vi "rsscope_core_global.vi"() -> ()   [LabVIEW 2014] (continued)
Name"="Protocol USB Trigger ET Check Max", "Data Type"=2, "Command"="TRIG{Trigger}:USB:TMAX", "Access"=2, "Range Table"="", "Read Callback"="", "Write Callback"="", "Supported Models"="", "Instrument Options"="K60", "Flags"=0, "Help"="Sets the end value of an endpoint type range if the corresponding condition is set to &apos;In range&apos; and &apos;Out of range&apos;.\n\nAvailable Repeated Capabilities:\nTrigger: TrigA, TrigB, TrigR\r\n\nRemote-control command(s):\nTRIGger<m>:USB:TMAX"}, {"Level"=2, "Class Only"=TRUE, "Identifier"="", "Descriptive Name"="USB 31 Generation 1", "Data Type"=0, "Command"="", "Access"=0, "Range Table"="", "Read Callback"="", "Write Callback"="", "Supported Models"="", "Instrument Options"="", "Flags"=0, "Help"="Configures USB 3.1 Generation 1 trigger."}, {"Level"=2, "Class Only"=TRUE, "Identifier"="", "Descriptive Name"="USB PD", "Data Type"=0, "Command"="", "Access"=0, "Range Table"="", "Read Callback"="", "Write Callback"="", "Supported Models"="", "Instrument Options"="", "Flags"=0, "Help"="Configures USB PD  trigger."}, {"Level"=3, "Class Only"=FALSE, "Identifier"="RSSCOPE_ATTR_USB_PD_TRIGGER_TYPE", "Descriptive Name"="USB PD Trigger Type", "Data Type"=0, "Command"="TRIG{Trigger}:USBP:TYPE", "Access"=2, "Range Table"="RsScope_rngUSBPDTriggerType", "Read Callback"="", "Write Callback"="", "Supported Models"="", "Instrument Options"="K63", "Flags"=0, "Help"="Selects the trigger type.\n\nAvailable Repeated Capabilities:\nTrigger: TrigA, TrigB, TrigR\r\n\nRemote-control command(s):\nTRIGger<m>:USBPd:TYPE"}, {"Level"=3, "Class Only"=FALSE, "Identifier"="RSSCOPE_ATTR_USB_PD_TRIGGER_PACKET_TYPE", "Descriptive Name"="USB PD Trigger Packet Type", "Data Type"=0, "Command"="TRIG{Trigger}:USBP:FRAM:SEL", "Access"=2, "Range Table"="RsScope_rngUSBPDPacketType", "Read Callback"="rsscope_empty_ReadCallback.vi", "Write Callback"="", "Supported Models"="", "Instrument Options"="K63", "Flags"=0, "Help"="Selects the frame to be triggered on, if the frame does not have any fields, e.g. a test frame.\n\nAvailable Repeated Capabilities:\nTrigger: TrigA, TrigB, TrigR\r\n\nRemote-control command(s):\nTRIGger<m>:USBPd:FRAMe:SELect"}, {"Level"=3, "Class Only"=TRUE, "Identifier"="", "Descriptive Name"="Data", "Data Type"=0, "Command"="", "Access"=0, "Range Table"="", "Read Callback"="", "Write Callback"="", "Supported Models"="", "Instrument Options"="", "Flags"=0, "Help"="Defines for the selected field, how a data check is executed."}, {"Level"=4, "Class Only"=FALSE, "Identifier"="RSSCOPE_ATTR_USB_PD_TRIGGER_DATA_CONDITION", "Descriptive Name"="USB PD Trigger Data Condition", "Data Type"=0, "Command"="TRIG{Trigger}:USBP:FRAM:FIEL{FieldNumber}:DOP", "Access"=2, "Range Table"="rsscope_rngProtocolTriggerCondition", "Read Callback"="rsscope_FormatUSBPDPacketTypeInt32_ReadCallback.vi", "Write Callback"="rsscope_FormatUSBPDPacketTypeInt32_WriteCallback.vi", "Supported Models"="", "Instrument Options"="K63", "Flags"=0, "Help"="Sets the condition for the data pattern. You can define no value, an exact value or a value range.\n\nAvailable Repeated Capabilities:\nTrigger: TrigA, TrigB, TrigR\r\nFieldNumber: Field1, Field2, Field3, Field4, Field5, Field6, Field7, Field8, Field9, Field10, Field11, Field12, Field13, Field14, Field15, Field16, Field17, Field18, Field19, Field20\r\n\nRemote-control command(s):\nTRIGger<m>:USBPd:FRAMe:FIELd<n>:DOPerator"}, {"Level"=4, "Class Only"=FALSE, "Identifier"="RSSCOPE_ATTR_USB_PD_TRIGGER_DATA_MIN", "Descriptive Name"="USB PD Trigger Data Min", "Data Type"=2, "Command"="TRIG{Trigger}:USBP:FRAM:FIEL{FieldNumber}:DMIN", "Access"=2, "Range Table"="", "Read Callback"="rsscope_FormatUSBPDPacketTypeString_ReadCallback.vi", "Write Callback"="rsscope_FormatUSBPDPacketTypeString_WriteCallback.vi", "Supported Models"="", "Instrument Options"="K63", "Flags"=0, "Help"="Specifies a data bit pattern, or sets the start value of a pattern range.\n\nValid Values:\nBinary pattern string consisting of 1; 0; or X (any bit).\n\nAvailable Repeated Capabilities:\nTrigger: TrigA, TrigB, TrigR\r\nFieldNumber: Field1, Field2, Field3, Field4, Field5, Field6, Field7, Field8, Field9, Field10, Field11, Field12, Field13, Field14, Field15, Field16, Field17, Field18, Field19, Field20\r\n\nRemote-control command(s):\nTRIGger<m>:USBPd:FRAMe:FIELd<n>:DMIN"}, {"Level"=4, "Class Only"=FALSE, "Identifier"="RSSCOPE_ATTR_USB_PD_TRIGGER_DATA_MAX", "Descriptive Name"="USB PD Trigger Data Max", "Data Type"=2, "Command"="TRIG{Trigger}:USBP:FRAM:FIEL{FieldNumber}:DMAX", "Access"=2, "Range Table"="", "Read Callback"="rsscope_FormatUSBPDPacketTypeString_ReadCallback.vi", "Write Callback"="rsscope_FormatUSBPDPacketTypeString_WriteCallback.vi", "Supported Models"="", "Instrument Options"="K63", "Flags"=0, "Help"="Sets the end value of a data type range for condition In Range or Out of Range. \n\nValid Values:\nBinary pattern string consisting of 1; 0; or X (any bit).\n\nAvailable Repeated Capabilities:\nTrigger: TrigA, TrigB, TrigR\r\nFieldNumber: Field1, Field2, Field3, Field4, Field5, Field6, Field7, Field8, Field9, Field10, Field11, Field12, Field13, Field14, Field15, Field16, Field17, Field18, Field19, Field20\r\n\nRemote-control command(s):\nTRIGger<m>:USBPd:FRAMe:FIELd<n>:DMAX"}, {"Level"=3, "Class Only"=TRUE, "Identifier"="", "Descriptive Name"="Index", "Data Type"=0, "Command"="", "Access"=0, "Range Table"="", "Read Callback"="", "Write Callback"="", "Supported Models"="", "Instrument Options"="", "Flags"=0, "Help"="Defines for the selected field, how an index check is executed."}, {"Level"=4, "Class Only"=FALSE, "Identifier"="RSSCOPE_ATTR_USB_PD_TRIGGER_INDEX_CONDITION", "Descriptive Name"="USB PD Trigger Index Condition", "Data Type"=0, "Command"="TRIG{Trigger}:USBP:FRAM:FIEL{FieldNumber}:IOP", "Access"=2, "Range Table"="rsscope_rngUSB31Gen1IndexCondition", "Read Callback"="rsscope_FormatUSBPDPacketTypeInt32_ReadCallback.vi", "Write Callback"="rsscope_FormatUSBPDPacketTypeInt32_WriteCallback.vi", "Supported Models"="", "Instrument Options"="K63", "Flags"=0, "Help"="Sets the operator for the index in the selected field of the selected frame.\n\nAvailable Repeated Capabilities:\nTrigger: TrigA, TrigB, TrigR\r\nFieldNumber: Field1, Field2, Field3, Field4, Field5, Field6, Field7, Field8, Field9, Field10, Field11, Field12, Field13, Field14, Field15, Field16, Field17, Field18, Field19, Field20\r\n\nRemote-control command(s):\nTRIGger<m>:USBPd:FRAMe:FIELd<n>:IOPerator"}, {"Level"=4, "Class Only"=FALSE, "Identifier"="RSSCOPE_ATTR_USB_PD_TRIGGER_INDEX_MIN", "Descriptive Name"="USB PD Trigger Index Min", "Data Type"=0, "Command"="TRIG{Trigger}:USBP:FRAM:FIEL{FieldNumber}:IMIN", "Access"=2, "Range Table"="", "Read Callback"="rsscope_FormatUSBPDPacketTypeInt32_ReadCallback.vi", "Write Callback"="rsscope_FormatUSBPDPacketTypeInt32_WriteCallback.vi", "Supported Models"="", "Instrument Options"="K63", "Flags"=0, "Help"="Specifies a data bit pattern, or sets the start value of a pattern range.\n\nValid Values:\nBinary pattern string consisting of 1; 0; or X (any bit).\n\nAvailable Repeated Capabilities:\nTrigger: TrigA, TrigB, TrigR\r\nFieldNumber: Field1, Field2, Field3, Field4, Field5, Field6, Field7, Field8, Field9, Field10, Field11, Field12, Field13, Field14, Field15, Field16, Field17, Field18, Field19, Field20\r\n\nRemote-control command(s):\nTRIGger<m>:USBPd:FRAMe:FIELd<n>:IMIN"}, {"Level"=4, "Class Only"=FALSE, "Identifier"="RSSCOPE_ATTR_USB_PD_TRIGGER_INDEX_MAX", "Descriptive Name"="USB PD Trigger Index Max", "Data Type"=0, "Command"="TRIG{Trigger}:USBP:FRAM:FIEL{FieldNumber}:IMAX", "Access"=2, "Range Table"="", "Read Callback"="rsscope_FormatUSBPDPacketTypeInt32_ReadCallback.vi", "Write Callback"="rsscope_FormatUSBPDPacketTypeInt32_WriteCallback.vi", "Supported Models"="", "Instrument Options"="K63", "Flags"=0, "Help"="Sets the end value of a data type range for condition In Range or Out of Range. \n\nValid Values:\nBinary pattern string consisting of 1; 0; or X (any bit).\n\nAvailable Repeated Capabilities:\nTrigger: TrigA, TrigB, TrigR\r\nFieldNumber: Field1, Field2, Field3, Field4, Field5, Field6, Field7, Field8, Field9, Field10, Field11, Field12, Field13, Field14, Field15, Field16, Field17, Field18, Field19, Field20\r\n\nRemote-control command(s):\nTRIGger<m>:USBPd:FRAMe:FIELd<n>:IMAX"}, {"Level"=3, "Class Only"=TRUE, "Identifier"="", "Descriptive Name"="Bit State", "Data Type"=0, "Command"="", "Access"=0, "Range Table"="", "Read Callback"="", "Write Callback"="", "Supported Models"="", "Instrument Options"="", "Flags"=0, "Help"="Defines the bit state to be checked for the selected field. Permitted bit states are 1, 0 or X (don&apos;t care)."}, {"Level"=4, "Class Only"=FALSE, "Identifier"="RSSCOPE_ATTR_USB_PD_TRIGGER_BIT_STATE", "Descriptive Name"="USB PD Trigger Bit State", "Data Type"=0, "Command"="TRIG{Trigger}:USBP:FRAM:FIEL{FieldNumber}:BIT", "Access"=2, "Range Table"="RsScope_rngBitState", "Read Callback"="rsscope_FormatUSBPDPacketTypeInt32_ReadCallback.vi", "Write Callback"="rsscope_FormatUSBPDPacketTypeInt32_WriteCallback.vi", "Supported Models"="", "Instrument Options"="K63", "Flags"=0, "Help"="Sets the bit state of a field that only consists of one bit.\n\nAvailable Repeated Capabilities:\nTrigger: TrigA, TrigB, TrigR\r\nFieldNumber: Field1, Field2, Field3, Field4, Field5, Field6, Field7, Field8, Field9, Field10, Field11, Field12, Field13, Field14, Field15, Field16, Field17, Field18, Field19, Field20\r\n\nRemote-control command(s):\nTRIGger<m>:USBPd:FRAMe:FIELd<n>:BIT"}, {"Level"=2, "Class Only"=TRUE, "Identifier"="", "Descriptive Name"="Custom Manchester NRZ", "Data Type"=0, "Command"="", "Access"=0, "Range Table"="", "Read Callback"="", "Write Callback"="", "Supported Models"="", "Instrument Options"="", "Flags"=0, "Help"="R&S RTO-K50 is a firmware option that enables the R&S RTO to analyze customizable serial bus signals encoded by the following coding standards: Manchester, Manchester II, NRZ Clocked, NRZ Unclocked."}, {"Level"=3, "Class Only"=FALSE, "Identifier"="RSSCOPE_ATTR_MANCHESTER_NRZ_TRIGGER_TYPE", "Descriptive Name"="Manchester NRZ Trigger Type", "Data Type"=0, "Command"="TRIG{Trigger}:CMSB:TYPE", "Access"=2, "Range Table"="RsScope_rngTriggerManchesterNRZType", "Read Callback"="", "Write Callback"="", "Supported Models"="", "Instrument Options"="K50", "Flags"=0, "Help"="Selects the trigger type for custom serial bus analysis.\n\nAvailable Repeated Capabilities:\nTrigger: TrigA, TrigB, TrigR\r\n\nRemote-control command(s):\nTRIGger<m>:CMSB:TYPE"}, {"Level"=3, "Class Only"=FALSE, "Identifier"="RSSCOPE_ATTR_MANCHESTER_NRZ_TRIGGER_DATA_PATTERN", "Descriptive Name"="Manchester NRZ Trigger Data Pattern", "Data Type"=2, "Command"="TRIG{Trigger}:CMSB:PATT", "Access"=2, "Range Table"="", "Read Callback"="", "Write Callback"="", "Supported Models"="", "Instrument Options"="K50", "Flags"=0, "Help"="Sets the pattern match conditions for a payload data check. The trigger is set to the first occurrence of a matching data bit pattern (which can be freely specified), starting after the minimum gap time and after the detected start of the data frame.\n\nAvailable Repeated Capabilities:\nTrigger: TrigA, TrigB, TrigR\r\n\nRemote-control command(s):\nTRIGger<m>:CMSB:PATTern"}, {"Level"=3, "Class Only"=FALSE, "Identifier"="RSSCOPE_ATTR_MANCHESTER_NRZ_TRIGGER_INDEX_CONDITION", "Descriptive Name"="Manchester NRZ Trigger Index Condition", "Data Type"=0, "Command"="TRIG{Trigger}:CMSB:ICON", "Access"=2, "Range Table"="rsscope_rngProtocolDataIndexOperator", "Read Callback"="", "Write Callback"="", "Supported Models"="", "Instrument Options"="K50", "Flags"=0, "Help"="Sets the operator to set a specific bit index (data position).\n\nAvailable Repeated Capabilities:\nTrigger: TrigA, TrigB, TrigR\r\n\nRemote-control command(s):\nTRIGger<m>:CMSB:ICONdition"}, {"Level"=3, "Class Only"=FALSE, "Identifier"="RSSCOPE_ATTR_MANCHESTER_NRZ_TRIGGER_INDEX_MIN", "Descriptive Name"="Manchester NRZ Trigger Index Min", "Data Type"=0, "Command"="TRIG{Trigger}:CMSB:IMIN", "Access"=2, "Range Table"="RsScope_rngManchesterNRZTriggerIndex", "Read Callback"="", "Write Callback"="", "Supported Models"="", "Instrument Options"="K50", "Flags"=0, "Help"="Sets the bit index (data position). If Index Condition is set to IN Range, IndexMin sets the start value of the bit index range.\n\nAvailable Repeated Capabilities:\nTrigger: TrigA, TrigB, TrigR\r\n\nRemote-control command(s):\nTRIGger<m>:CMSB:IMIN"}, {"Level"=3, "Class Only"=FALSE, "Identifier"="RSSCOPE_ATTR_MANCHESTER_NRZ_TRIGGER_INDEX_MAX", "Descriptive Name"="Manchester NRZ Trigger Index Max", "Data Type"=0, "Command"="TRIG{Trigger}:CMSB:IMAX", "Access"=2, "Range Table"="RsScope_rngManchesterNRZTriggerIndex", "Read Callback"="", "Write Callback"="", "Supported Models"="", "Instrument Options"="", "Flags"=0, "Help"="Sets the end value of the bit index range (data position range), if condition is set to In Range.\n\nAvailable Repeated Capabilities:\nTrigger: TrigA, TrigB, TrigR\r\n\nRemote-control command(s):\nTRIGger<m>:CMSB:IMAX"}, {"Level"=3, "Class Only"=FALSE, "Identifier"="RSSCOPE_ATTR_NRZ_TRIGGER_WORD_LENGTH", "Descriptive Name"="NRZ Trigger Word Length", "Data Type"=0, "Command"="TRIG{Trigger}:CMSB:NRZ:WRDL", "Access"=2, "Range Table"="RsScope_rngNRZTriggerWordLength", "Read Callback"="", "Write Callback"="", "Supported Models"="", "Instrument Options"="K50", "Flags"=0, "Help"="Sets the number of bits in an NRZ unclocked word.\n\nAvailable Repeated Capabilities:\nTrigger: TrigA, TrigB, TrigR\r\n\nRemote-control command(s):\nTRIGger<m>:CMSB:NRZ:WRDLength"}, {"Level"=2, "Class Only"=TRUE, "Identifier"="", "Descriptive Name"="SENT", "Data Type"=0, "Command"="", "Access"=0, "Range Table"="", "Read Callback"="", "Write Callback"="", "Supported Models"="", "Instrument Options"="", "Flags"=0, "Help"="SENT (Single Ended Nibble Transmission, R&S RTO-K10 option) is a serial transmission interface protocol originally specified for the communication of sensors and control units in automotive electronics."}, {"Level"=3, "Class Only"=FALSE, "Identifier"="RSSCOPE_ATTR_SENT_TRIGGER_TYPE", "Descriptive Name"="SENT Trigger Type", "Data Type"=0, "Command"="TRIG{Trigger}:SENT:TYPE", "Access"=2, "Range Table"="RsScope_rngSENTTriggerType", "Read Callback"="", "Write Callback"="", "Supported Models"="", "Instrument Options"="K10", "Flags"=0, "Help"="Selects the trigger event for the SENT transmission type.\n\nAvailable Repeated Capabilities:\nTrigger: TrigA, TrigB, TrigR\r\n\nRemote-control command(s):\nTRIGger<m>:SENT:TYPE"}, {"Level"=3, "Class Only"=TRUE, "Identifier"="", "Descriptive Name"="Transmission Sequence", "Data Type"=0, "Command"="", "Access"=0, "Range Table"="", "Read Callback"="", "Write Callback"="", "Supported Models"="", "Instrument Options"="", "Flags"=0, "Help"="Configures the trigger conditions for trigger type transmission sequence."}, {"Level"=4, "Class Only"=FALSE, "Identifier"="RSSCOPE_ATTR_SENT_TRIGGER_TRANSMISSION_SEQUENCE_TYPE", "Descriptive Name"="SENT Trigger Transmission Sequence Type", "Data Type"=0, "Command"="TRIG{Trigger}:SENT:TTYP", "Access"=2, "Range Table"="RsScope_rngSENTTriggerTSType", "Read Callback"="", "Write Callback"="", "Supported Models"="", "Instrument Options"="K10", "Flags"=0, "Help"="Selects the trigger event for the SENT transmission type.\n\nAvailable Repeated Capabilities:\nTrigger: TrigA, TrigB, TrigR\r\n\nRemote-control command(s):\nTRIGger<m>:SENT:TTYPe"}, {"Level"=4, "Class Only"=FALSE, "Identifier"="RSSCOPE_ATTR_SENT_TRIGGER_TRANSMISSION_SEQUENCE_STATUS", "Descriptive Name"="SENT Trigger Transmission Sequence Status", "Data Type"=2, "Command"="TRIG{Trigger}:SENT:STAT", "Access"=2, "Range Table"="", "Read Callback"="", "Write Callback"="", "Supported Models"="", "Instrument Options"="K10", "Flags"=0, "Help"="Sets the status nibble data, numeric or string pattern. The string parameter accepts the bit value X (don&apos;t care).\n\nAvailable Repeated Capabilities:\nTrigger: TrigA, TrigB, TrigR\r\n\nRemote-control command(s):\nTRIGger<m>:SENT:STATus"}, {"Level"=4, "Class Only"=FALSE, "Identifier"="RSSCOPE_ATTR_SENT_TRIGGER_TRANSMISSION_SEQUENCE_CONDITION", "Descriptive Name"="SENT Trigger Transmission Sequence Condition", "Data Type"=0, "Command"="TRIG{Trigger}:SENT:TDCN", "Access"=2, "Range Table"="rsscope_rngProtocolTriggerCondition", "Read Callback"="", "Write Callback"="", "Supported Models"="", "Instrument Options"="K10", "Flags"=0, "Help"="Sets the operator to set a specific data pattern or a data pattern range.\n\nAvailable Repeated Capabilities:\nTrigger: TrigA, TrigB, TrigR\r\n\nRemote-control command(s):\nTRIGger<m>:SENT:TDCN"}, {"Level"=4, "Class Only"=FALSE, "Identifier"="RSSCOPE_ATTR_SENT_TRIGGER_TRANSMISSION_SEQUENCE_DATA_MIN", "Descriptive Name"="SENT Trigger Transmission Sequence Data Min", "Data Type"=2, "Command"="TRIG{Trigger}:SENT:TDMN", "Access"=2, "Range Table"="", "Read Callback"="", "Write Callback"="", "Supported Models"="", "Instrument Options"="K10", "Flags"=0, "Help"="Specifies a data pattern, or sets the start value of a data pattern range. \n\nValid Values:\nBinary pattern string consisting of 1; 0; or X (any bit).\n\nAvailable Repeated Capabilities:\nTrigger: TrigA, TrigB, TrigR\r\n\nRemote-control command(s):\nTRIGger<m>:SENT:TDMN"}, {"Level"=4, "Class Only"=FALSE, "Identifier"="RSSCOPE_ATTR_SENT_TRIGGER_TRANSMISSION_SEQUENCE_DATA_MAX", "Descriptive Name"="SENT Trigger Transmission Sequence Data Max", "Data Type"=2, "Command"="TRIG{Trigger}:SENT:TDMX", "Access"=2, "Range Table"="", "Read Callback"="", "Write Callback"="", "Supported Models"="", "Instrument Options"="K10", "Flags"=0, "Help"="Sets the end value of an identifier range for condition In Range or Out of Range. \n\nValid Values:\nBinary pattern string consisting of 1; 0; or X (any bit).\n\nAvailable Repeated Capabilities:\nTrigger: TrigA, TrigB, TrigR\r\n\nRemote-control command(s):\nTRIGger<m>:SENT:TDMX"}, {"Level"=3, "Class Only"=TRUE, "Identifier"="", "Descriptive Name"="Serial Message", "Data Type"=0, "Command"="", "Access"=0, "Range Table"="", "Read Callback"="", "Write Callback"="", "Supported Models"="", "Instrument Options"="", "Flags"=0, "Help"="Configures the trigger conditions for a serial message."}, {"Level"=4, "Class Only"=FALSE, "Identifier"="RSSCOPE_ATTR_SENT_TRIGGER_SERIAL_MESSAGE_TYPE", "Descriptive Name"="SENT Trigger Serial Message Type", "Data Type"=0, "Command"="TRIG{Trigger}:SENT:STYP", "Access"=2, "Range Table"="RsScope_rngSENTTriggerSMType", "Read Callback"="", "Write Callback"="", "Supported Models"="", "Instrument Options"="K10", "Flags"=0, "Help"="Selects the trigger event for the serial message.\n\nAvailable Repeated Capabilities:\nTrigger: TrigA, TrigB, TrigR\r\n\nRemote-control command(s):\nTRIGger<m>:SENT:STYPe"}, {"Level"=4, "Class Only"=FALSE, "Identifier"="RSSCOPE_ATTR_SENT_TRIGGER_SERIAL_MESSAGE_ID_TYPE", "Descriptive Name"="SENT Trigger Serial Message ID Type", "Data Type"=0, "Command"="TRIG{Trigger}:SENT:SIDT", "Access"=2, "Range Table"="RsScope_rngSENTIDType", "Read Callback"="", "Write Callback"="", "Supported Models"="", "Instrument Options"="K10", "Flags"=0, "Help"="Sets the message ID format (4 bit or 8 bit) of the enhanced serial message.\n\nAvailable Repeated Capabilities:\nTrigger: TrigA, TrigB, TrigR\r\n\nRemote-control command(s):\nTRIGger<m>:SENT:SIDType"}, {"Level"=4, "Class Only"=FALSE, "Identifier"="RSSCOPE_ATTR_SENT_TRIGGER_SERIAL_MESSAGE_ID_CONDITION", "Descriptive Name"="SENT Trigger Serial Message ID Condition", "Data Type"=0, "Command"="TRIG{Trigger}:SENT:SICN", "Access"=2, "Range Table"="rsscope_rngProtocolTriggerCondition", "Read Callback"="", "Write Callback"="", "Supported Models"="", "Instrument Options"="K10", "Flags"=0, "Help"="Sets the operator to set a specific data pattern or a data pattern range.\n\nAvailable Repeated Capabilities:\nTrigger: TrigA, TrigB, TrigR\r\n\nRemote-control command(s):\nTRIGger<m>:SENT:SICN"}, {"Level"=4, "Class Only"=FALSE, "Identifier"="RSSCOPE_ATTR_SENT_TRIGGER_SERIAL_MESSAGE_ID_MIN", "Descriptive Name"="SENT Trigger Serial Message ID Min", "Data Type"=2, "Command"="TRIG{Trigger}:SENT:SIMN", "Access"=2, "Range Table"="", "Read Callback"="", "Write Callback"="", "Supported Models"="", "Instrument Options"="K10", "Flags"=0, "Help"="Specifies a message identifier pattern, or sets the start value of an identifier range. \n\nValid Values:\nBinary pattern string consisting of 1; 0; or X (any bit).\n\nAvailable Repeated Capabilities:\nTrigger: TrigA, TrigB, TrigR\r\n\nRemote-control command(s):\nTRIGger<m>:SENT:SIMN"}, {"Level"=4, "Class Only"=FALSE, "Identifier"="RSSCOPE_ATTR_SENT_TRIGGER_SERIAL_MESSAGE_ID_MAX", "Descriptive Name"="SENT Trigger Serial Message ID Max", "Data Type"=2, "Command"="TRIG{Trigger}:SENT:SIMX", "Access"=2, "Range Table"="", "Read Callback"="", "Write Callback"="", "Supported Models"="", "Instrument Options"="K10", "Flags"=0, "Help"="Sets the end value of an identifier range for condition In Range or Out of Range.\n\nValid Values:\nBinary pattern string consisting of 1; 0; or X (any bit).\n\nAvailable Repeated Capabilities:\nTrigger: TrigA, TrigB, TrigR\r\n\nRemote-control command(s):\nTRIGger<m>:SENT:SIMX"}, {"Level"=4, "Class Only"=FALSE, "Identifier"="RSSCOPE_ATTR_SENT_TRIGGER_SERIAL_MESSAGE_DATA_CONDITION", "Descriptive Name"="SENT Trigger Serial Message Data Condition", "Data Type"=0, "Command"="TRIG{Trigger}:SENT:SDCN", "Access"=2, "Range Table"="rsscope_rngProtocolTriggerCondition", "Read Callback"="", "Write Callback"="", "Supported Models"="", "Instrument Options"="K10", "Flags"=0, "Help"="Sets the operator to define a specific data pattern or a data pattern range.\n\nAvailable Repeated Capabilities:\nTrigger: TrigA, TrigB, TrigR\r\n\nRemote-control command(s):\nTRIGger<m>:SENT:SDCN"}, {"Level"=4, "Class Only"=FALSE, "Identifier"="RSSCOPE_ATTR_SENT_TRIGGER_SERIAL_MESSAGE_DATA_MIN", "Descriptive Name"="SENT Trigger Serial Message Data Min", "Data Type"=2, "Command"="TRIG{Trigger}:SENT:SDMN", "Access"=2, "Range Table"="", "Read Callback"="", "Write Callback"="", "Supported Models"="", "Instrument Options"="K10", "Flags"=0, "Help"="Specifies a data pattern, or sets the start value of a data pattern range.\n\nValid Values:\nBinary pattern string consisting of 1; 0; or X (any bit).\n\nAvailable Repeated Capabilities:\nTrigger: TrigA, TrigB, TrigR\r\n\nRemote-control command(s):\nTRIGger<m>:SENT:SDMN"}, {"Level"=4, "Class Only"=FALSE, "Identifier"="RSSCOPE_ATTR_SENT_TRIGGER_SERIAL_MESSAGE_DATA_MAX", "Descriptive Name"="SENT Trigger Serial Message Data Max", "Data Type"=2, "Command"="TRIG{Trigger}:SENT:SDMX", "Access"=2, "Range Table"="", "Read Callback"="", "Write Callback"="", "Supported Models"="", "Instrument Options"="K10", "Flags"=0, "Help"="Sets the end value of an identifier range for condition In Range or Out of Range.\n\nValid Values:\nBinary pattern string consisting of 1; 0; or X (any bit).\n\nAvailable Repeated Capabilities:\nTrigger: TrigA, TrigB, TrigR\r\n\nRemote-control command(s):\nTRIGger<m>:SENT:SDMX"}, {"Level"=3, "Class Only"=TRUE, "Identifier"="", "Descriptive Name"="Error Conditions", "Data Type"=0, "Command"="", "Access"=0, "Range Table"="", "Read Callback"="", "Write Callback"="", "Supported Models"="", "Instrument Options"="", "Flags"=0, "Help"="This class configures conditions for Error trigger."}, {"Level"=4, "Class Only"=FALSE, "Identifier"="RSSCOPE_ATTR_PROTOCOL_SENT_TRIGGER_FORM_ERROR", "Descriptive Name"="Protocol SENT Trigger Form Error", "Data Type"=3, "Command"="TRIG{Trigger}:SENT:FORM", "Access"=2, "Range Table"="", "Read Callback"="", "Write Callback"="", "Supported Models"="", "Instrument Options"="K10", "Flags"=0, "Help"="Triggers on format errors in serial messages.\n\nAvailable Repeated Capabilities:\nTrigger: TrigA, TrigB, TrigR\r\n\nRemote-control command(s):\nTRIGger<m>:SENT:FORMerror"}, {"Level"=4, "Class Only"=FALSE, "Identifier"="RSSCOPE_ATTR_PROTOCOL_SENT_TRIGGER_CALIBRATION_PULSE_ERROR", "Descriptive Name"="Protocol SENT Trigger Calibration Pulse Error", "Data Type"=3, "Command"="TRIG{Trigger}:SENT:PULS", "Access"=2, "Range Table"="", "Read Callback"="", "Write Callback"="", "Supported Models"="", "Instrument Options"="K10", "Flags"=0, "Help"="Triggers on calibration pulse erors in transmission sequences.\n\nAvailable Repeated Capabilities:\nTrigger: TrigA, TrigB, TrigR\r\n\nRemote-control command(s):\nTRIGger<m>:SENT:PULSeerror"}, {"Level"=4, "Class Only"=FALSE, "Identifier"="RSSCOPE_ATTR_PROTOCOL_SENT_TRIGGER_PULSE_PERIOD_ERROR", "Descriptive Name"="Protocol SENT Trigger Pulse Period Error", "Data Type"=3, "Command"="TRIG{Trigger}:SENT:PPER", "Access"=2, "Range Table"="", "Read Callback"="", "Write Callback"="", "Supported Models"="", "Instrument Options"="K10", "Flags"=0, "Help"="Triggers on pulse period errors.\n\nAvailable Repeated Capabilities:\nTrigger: TrigA, TrigB, TrigR\r\n\nRemote-control command(s):\nTRIGger<m>:SENT:PPERioderror"}, {"Level"=4, "Class Only"=FALSE, "Identifier"="RSSCOPE_ATTR_PROTOCOL_SENT_TRIGGER_CRC_ERROR", "Descriptive Name"="Protocol SENT Trigger CRC Error", "Data Type"=3, "Command"="TRIG{Trigger}:SENT:CRC", "Access"=2, "Range Table"="", "Read Callback"="", "Write Callback"="", "Supported Models"="", "Instrument Options"="K10", "Flags"=0, "Help"="Triggers on CRC errors in both, the transmission sequences and serial messages.\n\nAvailable Repeated Capabilities:\nTrigger: TrigA, TrigB, TrigR\r\n\nRemote-control command(s):\nTRIGger<m>:SENT:CRCerror"}, {"Level"=4, "Class Only"=FALSE, "Identifier"="RSSCOPE_ATTR_PROTOCOL_SENT_TRIGGER_IRREGULAR_FRAME_LENGTH_ERROR", "Descriptive Name"="Protocol SENT Trigger Irregular Frame Length Error", "Data Type"=3, "Command"="TRIG{Trigger}:SENT:IRFL", "Access"=2, "Range Table"="", "Read Callback"="", "Write Callback"="", "Supported Models"="", "Instrument Options"="K10", "Flags"=0, "Help"="Triggers on frame length errors in transmission sequences when pause pulse for constant frame length is set.\n\nAvailable Repeated Capabilities:\nTrigger: TrigA, TrigB, TrigR\r\n\nRemote-control command(s):\nTRIGger<m>:SENT:IRFLength"}, {"Level"=2, "Class Only"=TRUE, "Identifier"="", "Descriptive Name"="D-PHY", "Data Type"=0, "Command"="", "Access"=0, "Range Table"="", "Read Callback"="", "Write Callback"="", "Supported Models"="", "Instrument Options"="", "Flags"=0, "Help"="In this class all trigger settings can be configured."}, {"Level"=3, "Class Only"=FALSE, "Identifier"="RSSCOPE_ATTR_DPHY_TRIGGER_TYPE", "Descriptive Name"="DPHY Trigger Type", "Data Type"=0, "Command"="TRIG{Trigger}:DPHY:TYPE", "Access"=2, "Range Table"="RsScope_rngDPHYTriggerType", "Read Callback"="", "Write Callback"="", "Supported Models"="", "Instrument Options"="K42", "Flags"=0, "Help"="Sets the type of frame to be triggered on.\n\nAvailable Repeated Capabilities:\nTrigger: TrigA, TrigB, TrigR\r\n\nRemote-control command(s):\nTRIGger<m>:DPHY:TYPE"}, {"Level"=3, "Class Only"=FALSE, "Identifier"="RSSCOPE_ATTR_DPHY_TRIGGER_VIRTUAL_CHANNEL", "Descriptive Name"="DPHY Trigger Virtual Channel", "Data Type"=2, "Command"="TRIG{Trigger}:DPHY:HSVC", "Access"=2, "Range Table"="", "Read Callback"="", "Write Callback"="", "Supported Models"="", "Instrument Options"="K42", "Flags"=0, "Help"="Sets the virtual channel to be triggered on.\n\nAvailable Repeated Capabilities:\nTrigger: TrigA, TrigB, TrigR\r\n\nRemote-control command(s):\nTRIGger<m>:DPHY:HSVC"}, {"Level"=3, "Class Only"=TRUE, "Identifier"="", "Descriptive Name"="Data Type", "Data Type"=0, "Command"="", "Access"=0, "Range Table"="", "Read Callback"="", "Write Callback"="", "Supported Models"="", "Instrument Options"="", "Flags"=0, "Help"="Sets the specified data type to be triggered on. The data type setup consists of the condition and one or two data patterns."}, {"Level"=4, "Class Only"=FALSE, "Identifier"="RSSCOPE_ATTR_DPHY_TRIGGER_DATA_TYPE_CONDITION", "Descriptive Name"="DPHY Trigger Data Type Condition", "Data Type"=0, "Command"="TRIG{Trigger}:DPHY:DTYP:COND", "Access"=2, "Range Table"="rsscope_rngProtocolTriggerCondition", "Read Callback"="", "Write Callback"="", "Supported Models"="", "Instrument Options"="K42", "Flags"=0, "Help"="Set the condition for the data type. You can define an exact value or a value range.\n\nAvailable Repeated Capabilities:\nTrigger: TrigA, TrigB, TrigR\r\n\nRemote-control command(s):\nTRIGger<m>:DPHY:DTYPe:CONDition"}, {"Level"=4, "Class Only"=FALSE, "Identifier"="RSSCOPE_ATTR_DPHY_TRIGGER_DATA_TYPE_MIN", "Descriptive Name"="DPHY Trigger Data Type Min", "Data Type"=2, "Command"="TRIG{Trigger}:DPHY:DTYP:MIN", "Access"=2, "Range Table"="", "Read Callback"="", "Write Callback"="", "Supported Models"="", "Instrument Options"="K42", "Flags"=0, "Help"="Specifies a data type pattern, or sets the start value of a pattern range.\n\nValid Values:\nBinary pattern string consisting of 1; 0; or X (any bit).\n\nAvailable Repeated Capabilities:\nTrigger: TrigA, TrigB, TrigR\r\n\nRemote-control command(s):\nTRIGger<m>:DPHY:DTYPe:MIN"}, {"Level"=4, "Class Only"=FALSE, "Identifier"="RSSCOPE_ATTR_DPHY_TRIGGER_DATA_TYPE_MAX", "Descriptive Name"="DPHY Trigger Data Type Max", "Data Type"=2, "Command"="TRIG{Trigger}:DPHY:DTYP:MAX", "Access"=2, "Range Table"="", "Read Callback"="", "Write Callback"="", "Supported Models"="", "Instrument Options"="K42", "Flags"=0, "Help"="Sets the end value of a data type range for condition In Range or Out of Range. \n\nValid Values:\nBinary pattern string consisting of 1; 0; or X (any bit).\n\nAvailable Repeated Capabilities:\nTrigger: TrigA, TrigB, TrigR\r\n\nRemote-control command(s):\nTRIGger<m>:DPHY:DTYPe:MAX"}, {"Level"=3, "Class Only"=TRUE, "Identifier"="", "Descriptive Name"="Word Count", "Data Type"=0, "Command"="", "Access"=0, "Range Table"="", "Read Callback"="", "Write Callback"="", "Supported Models"="", "Instrument Options"="", "Flags"=0, "Help"="Sets the specified data type to be triggered on. The word count setup consists of the condition and one or two data patterns."}, {"Level"=4, "Class Only"=FALSE, "Identifier"="RSSCOPE_ATTR_DPHY_TRIGGER_WORD_COUNT_CONDITION", "Descriptive Name"="DPHY Trigger Word Count Condition", "Data Type"=0, "Command"="TRIG{Trigger}:DPHY:WCO:COND", "Access"=2, "Range Table"="rsscope_rngProtocolTriggerCondition", "Read Callback"="", "Write Callback"="", "Supported Models"="", "Instrument Options"="K42", "Flags"=0, "Help"="Set the condition for the word count. You can define an exact value or a value range.\n\nAvailable Repeated Capabilities:\nTrigger: TrigA, TrigB, TrigR\r\n\nRemote-control command(s):\nTRIGger<m>:DPHY:WCOunt:CONDition"}, {"Level"=4, "Class Only"=FALSE, "Identifier"="RSSCOPE_ATTR_DPHY_TRIGGER_WORD_COUNT_MIN", "Descriptive Name"="DPHY Trigger Word Count Min", "Data Type"=2, "Command"="TRIG{Trigger}:DPHY:WCO:MIN", "Access"=2, "Range Table"="", "Read Callback"="", "Write Callback"="", "Supported Models"="", "Instrument Options"="K42", "Flags"=0, "Help"="Specifies a word bit pattern, or sets the start value of a pattern range.\n\nValid Values:\nBinary pattern string consisting of 1; 0; or X (any bit).\n\nAvailable Repeated Capabilities:\nTrigger: TrigA, TrigB, TrigR\r\n\nRemote-control command(s):\nTRIGger<m>:DPHY:WCOunt:MIN"}, {"Level"=4, "Class Only"=FALSE, "Identifier"="RSSCOPE_ATTR_DPHY_TRIGGER_WORD_COUNT_MAX", "Descriptive Name"="DPHY Trigger Word Count Max", "Data Type"=2, "Command"="TRIG{Trigger}:DPHY:WCO:MAX", "Access"=2, "Range Table"="", "Read Callback"="", "Write Callback"="", "Supported Models"="", "Instrument Options"="K42", "Flags"=0, "Help"="Sets the end value of a data type range for condition In Range or Out of Range. \n\nValid Values:\nBinary pattern string consisting of 1; 0; or X (any bit).\n\nAvailable Repeated Capabilities:\nTrigger: TrigA, TrigB, TrigR\r\n\nRemote-control command(s):\nTRIGger<m>:DPHY:WCOunt:MAX"}, {"Level"=3, "Class Only"=TRUE, "Identifier"="", "Descriptive Name"="Data", "Data Type"=0, "Command"="", "Access"=0, "Range Table"="", "Read Callback"="", "Write Callback"="", "Supported Models"="", "Instrument Options"="", "Flags"=0, "Help"="Set the specified data value to be triggered on.The data value setup consists of the\ncondition and one or two data value patterns."}, {"Level"=4, "Class Only"=FALSE, "Identifier"="RSSCOPE_ATTR_DPHY_TRIGGER_HIGH_SPEED_DATA_CONDITION", "Descriptive Name"="DPHY Trigger High Speed Data Condition", "Data Type"=0, "Command"="TRIG{Trigger}:DPHY:DATA:COND", "Access"=2, "Range Table"="rsscope_rngProtocolTriggerCondition", "Read Callback"="", "Write Callback"="", "Supported Models"="", "Instrument Options"="K42", "Flags"=0, "Help"="Set the condition for the data value. You can define an exact value or a value range.\n\nAvailable Repeated Capabilities:\nTrigger: TrigA, TrigB, TrigR\r\n\nRemote-control command(s):\nTRIGger<m>:DPHY:DATA:CONDition"}, {"Level"=4, "Class Only"=FALSE, "Identifier"="RSSCOPE_ATTR_DPHY_TRIGGER_HIGH_SPEED_DATA_MIN", "Descriptive Name"="DPHY Trigger High Speed Data Min", "Data Type"=2, "Command"="TRIG{Trigger}:DPHY:DATA:MIN", "Access"=2, "Range Table"="", "Read Callback"="", "Write Callback"="", "Supported Models"="", "Instrument Options"="K42", "Flags"=0, "Help"="Specifies a data bit pattern, or sets the start value of a pattern range.\n\nValid Values:\nBinary pattern string consisting of 1; 0; or X (any bit).\n\nAvailable Repeated Capabilities:\nTrigger: TrigA, TrigB, TrigR\r\n\nRemote-control command(s):\nTRIGger<m>:DPHY:DATA:MIN"}, {"Level"=4, "Class Only"=FALSE, "Identifier"="RSSCOPE_ATTR_DPHY_TRIGGER_HIGH_SPEED_DATA_MAX", "Descriptive Name"="DPHY Trigger High Speed Data Max", "Data Type"=2, "Command"="TRIG{Trigger}:DPHY:DATA:MAX", "Access"=2, "Range Table"="", "Read Callback"="", "Write Callback"="", "Supported Models"="", "Instrument Options"="K42", "Flags"=0, "Help"="Sets the end value of a data type range for condition In Range or Out of Range. \n\nValid Values:\nBinary pattern string consisting of 1; 0; or X (any bit).\n\nAvailable Repeated Capabilities:\nTrigger: TrigA, TrigB, TrigR\r\n\nRemote-control command(s):\nTRIGger<m>:DPHY:DATA:MAX"}, {"Level"=4, "Class Only"=FALSE, "Identifier"="RSSCOPE_ATTR_DPHY_TRIGGER_LOW_POWER_ESCAPE_MODE_DATA_CONDITION", "Descriptive Name"="DPHY Trigger Low Power Escape Mode Data Condition", "Data Type"=0, "Command"="TRIG{Trigger}:DPHY:ESDT:COND", "Access"=2, "Range Table"="rsscope_rngProtocolTriggerCondition", "Read Callback"="", "Write Callback"="", "Supported Models"="", "Instrument Options"="K42", "Flags"=0, "Help"="Set the condition for the escape mode data value. You can define an exact value or a value range.\n\nAvailable Repeated Capabilities:\nTrigger: TrigA, TrigB, TrigR\r\n\nRemote-control command(s):\nTRIGger<m>:DPHY:ESDTa:CONDition"}, {"Level"=4, "Class Only"=FALSE, "Identifier"="RSSCOPE_ATTR_DPHY_TRIGGER_LOW_POWER_ESCAPE_MODE_DATA_MIN", "Descriptive Name"="DPHY Trigger Low Power Escape Mode Data Min", "Data Type"=2, "Command"="TRIG{Trigger}:DPHY:ESDT:MIN", "Access"=2, "Range Table"="", "Read Callback"="", "Write Callback"="", "Supported Models"="", "Instrument Options"="K42", "Flags"=0, "Help"="Specifies an escape mode data bit pattern, or sets the start value of a pattern range.\n\nValid Values:\nBinary pattern string consisting of 1; 0; or X (any bit).\n\nAvailable Repeated Capabilities:\nTrigger: TrigA, TrigB, TrigR\r\n\nRemote-control command(s):\nTRIGger<m>:DPHY:ESDTa:MIN"}, {"Level"=4, "Class Only"=FALSE, "Identifier"="RSSCOPE_ATTR_DPHY_TRIGGER_LOW_POWER_ESCAPE_MODE_DATA_MAX", "Descriptive Name"="DPHY Trigger Low Power Escape Mode Data Max", "Data Type"=2, "Command"="TRIG{Trigger}:DPHY:ESDT:MAX", "Access"=2, "Range Table"="", "Read Callback"="", "Write Callback"="", "Supported Models"="", "Instrument Options"="K42", "Flags"=0, "Help"="Sets the end value of a escape mode data type range for condition In Range or Out of Range. \n\nValid Values:\nBinary pattern string consisting of 1; 0; or X (any bit).\n\nAvailable Repeated Capabilities:\nTrigger: TrigA, TrigB, TrigR\r\n\nRemote-control command(s):\nTRIGger<m>:DPHY:ESDTa:MAX"}, {"Level"=3, "Class Only"=TRUE, "Identifier"="", "Descriptive Name"="Data Index", "Data Type"=0, "Command"="", "Access"=0, "Range Table"="", "Read Callback"="", "Write Callback"="", "Supported Models"="", "Instrument Options"="", "Flags"=0, "Help"="Data index sets the range within this series of the data value that is considered for the analysis. The data index setup consists of the condition and one or two data index values."}, {"Level"=4, "Class Only"=FALSE, "Identifier"="RSSCOPE_ATTR_DPHY_TRIGGER_HIGH_SPEED_DATA_INDEX_CONDITION", "Descriptive Name"="DPHY Trigger High Speed Data Index Condition", "Data Type"=0, "Command"="TRIG{Trigger}:DPHY:DIDX:COND", "Access"=2, "Range Table"="rsscope_rngProtocolTriggerCondition", "Read Callback"="", "Write Callback"="", "Supported Models"="", "Instrument Options"="K42", "Flags"=0, "Help"="Sets the condition for the data index. You can define an exact value or a value range.\n\nAvailable Repeated Capabilities:\nTrigger: TrigA, TrigB, TrigR\r\n\nRemote-control command(s):\nTRIGger<m>:DPHY:DIDX:CONDition"}, {"Level"=4, "Class Only"=FALSE, "Identifier"="RSSCOPE_ATTR_DPHY_TRIGGER_HIGH_SPEED_DATA_INDEX_MIN", "Descriptive Name"="DPHY Trigger High Speed Data Index Min", "Data Type"=0, "Command"="TRIG{Trigger}:DPHY:DIDX:MIN", "Access"=2, "Range Table"="", "Read Callback"="", "Write Callback"="", "Supported Models"="", "Instrument Options"="K42", "Flags"=0, "Help"="Specifies a data index minimum, or sets the start value of a range.\n\nAvailable Repeated Capabilities:\nTrigger: TrigA, TrigB, TrigR\r\n\nRemote-control command(s):\nTRIGger<m>:DPHY:DIDX:MIN"}, {"Level"=4, "Class Only"=FALSE, "Identifier"="RSSCOPE_ATTR_DPHY_TRIGGER_HIGH_SPEED_DATA_INDEX_MAX", "Descriptive Name"="DPHY Trigger High Speed Data Index Max", "Data Type"=0, "Command"="TRIG{Trigger}:DPHY:DIDX:MAX", "Access"=2, "Range Table"="", "Read Callback"="", "Write Callback"="", "Supported Models"="", "Instrument Options"="K42", "Flags"=0, "Help"="Sets the end value of a data index range for condition In Range or Out of Range.\n\nAvailable Repeated Capabilities:\nTrigger: TrigA, TrigB, TrigR\r\n\nRemote-control command(s):\nTRIGger<m>:DPHY:DIDX:MAX"}, {"Level"=4, "Class Only"=FALSE, "Identifier"="RSSCOPE_ATTR_DPHY_TRIGGER_LOW_POWER_ESCAPE_MODE_DATA_INDEX_CONDITION", "Descriptive Name"="DPHY Trigger Low Power Escape Mode Data Index Condition", "Data Type"=0, "Command"="TRIG{Trigger}:DPHY:ESIN:COND", "Access"=2, "Range Table"="rsscope_rngProtocolTriggerCondition", "Read Callback"="", "Write Callback"="", "Supported Models"="", "Instrument Options"="K42", "Flags"=0, "Help"="Sets the condition for the escape mode data index. You can define an exact value or a value range.\n\nAvailable Repeated Capabilities:\nTrigger: TrigA, TrigB, TrigR\r\n\nRemote-control command(s):\nTRIGger<m>:DPHY:ESINdex:CONDition"}, {"Level"=4, "Class Only"=FALSE, "Identifier"="RSSCOPE_ATTR_DPHY_TRIGGER_LOW_POWER_ESCAPE_MODE_DATA_INDEX_MIN", "Descriptive Name"="DPHY Trigger Low Power Escape Mode Data Index Min", "Data Type"=0, "Command"="TRIG{Trigger}:DPHY:ESIN:MIN", "Access"=2, "Range Table"="", "Read Callback"="", "Write Callback"="", "Supported Models"="", "Instrument Options"="K42", "Flags"=0, "Help"="Specifies an escape mode data index minimum, or sets the start value of a range.\n\nAvailable Repeated Capabilities:\nTrigger: TrigA, TrigB, TrigR\r\n\nRemote-control command(s):\nTRIGger<m>:DPHY:ESINdex:MIN"}, {"Level"=4, "Class Only"=FALSE, "Identifier"="RSSCOPE_ATTR_DPHY_TRIGGER_LOW_POWER_ESCAPE_MODE_DATA_INDEX_MAX", "Descriptive Name"="DPHY Trigger Low Power Escape Mode Data Index Max", "Data Type"=0, "Command"="TRIG{Trigger}:DPHY:ESIN:MAX", "Access"=2, "Range Table"="", "Read Callback"="", "Write Callback"="", "Supported Models"="", "Instrument Options"="K42", "Flags"=0, "Help"="Sets the end value of a data index range for 
